vi "Add to composition.vi"(6 "Gate name":string, 9 "Wire depth":i32, 10 "Wire No":i32, 11 "Composition in":string[][](array[string])) -> (3 "Composition out":string[][](array[string]))   [LabVIEW 2016]
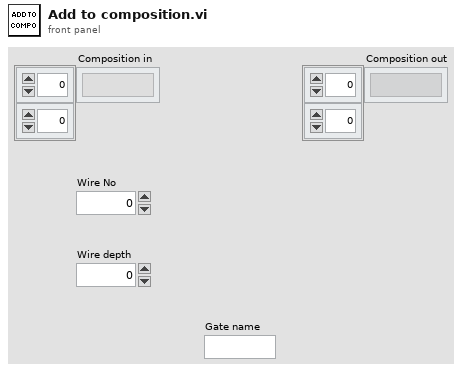
[diagram p1: front panel]
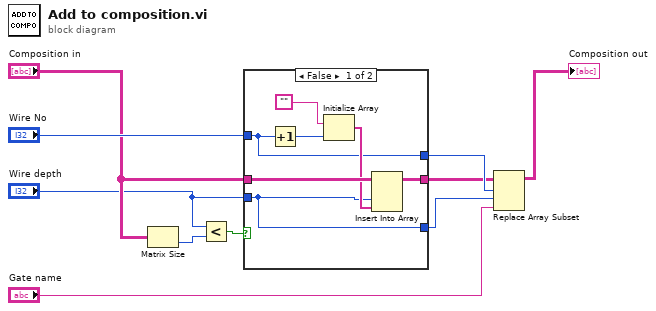
[diagram p0: block diagram]
diagram:
  n1 = Matrix Size(0:"Composition in") -> (2:w2:i32)  [unwired: 1 out]
  n2 = Less?(x="Wire depth", y=w2) -> (x < y?=w1:bool)
  n3 = case shown="False" w1 {
    tunnel: "Wire depth" -> [w12 w19]
    tunnel: "Composition in" -> [w17 w20]
    tunnel: [w14 w20] -> w7
    tunnel: [w12 w19] -> w10
    tunnel: [w11 w18] -> w9
    tunnel: "Wire No" -> [w11 w18]
    frame False {
      n4 = Increment(x=w11) -> (x+1=w13:i32)
      n5 = Initialize Array("", w13) -> (w15:string[])
      n6 = Insert Into Array(array=w17, index (col)=w12, new element=w15) -> (w14:string[][])  [unwired: 1 in]
    }
    frame True {
    }
  }
  n7 = Replace Array Subset(array=w7, new element="Gate name", index (row)=w9, index (col)=w10) -> (→"Composition out":string[][])
